vi "Define Target.vi"(8 "error in (no error)":errorcluster, 10 "Target Enqueuer ID":string, 11 "Targetted Msg in":refnum<class "Addressed Msg.lvclass">) -> (0 "error out":errorcluster, 3 "Targetted Msg out":refnum<class "Addressed Msg.lvclass">)   [LabVIEW 2020, in "Publisher.lvlib" / "Addressed Msg.lvclass"]
doc: "Configure 'Addressed Msg' for execution."
uses:
  Addressed Msg.lvclass
  Addressed Msg.lvclass/Addressed Msg.ctl
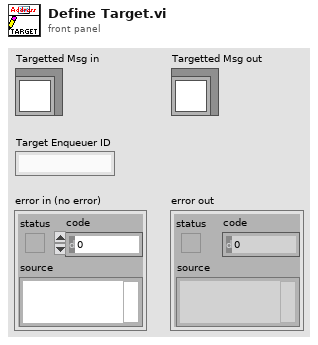
[diagram p1: front panel]
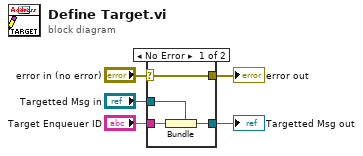
[diagram p0: block diagram]
diagram:
  n1 = case shown="No Error" "error in (no error)" {
    selector: "error in (no error)" -> [w7 w10]
    tunnel: [w7 w10] -> w4
    tunnel: [w9 w11] -> w2
    tunnel: "Targetted Msg in" -> [w6 w11]
    tunnel: "Target Enqueuer ID" -> [w8 _]
    frame No Error {
      n2 = Bundle(cluster=w6, w8) -> (w9:refnum<class "Addressed Msg.lvclass">)
    }
    frame Error {
    }
  }
  "error out" <- w4
  "Targetted Msg out" <- w2
